vi "Get_New_Path_from_raw_data.vi"(9 "New Results File Name":string, 10 "New Results Folder Name":string, 11 "Raw data file":path) -> (2 "Does it already exist?":bool, 3 "New Spreadsheet Results File":path)   [LabVIEW 2011]
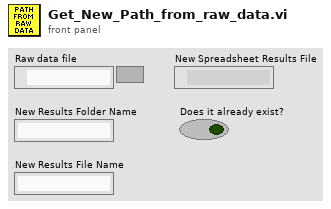
[diagram p1: front panel]
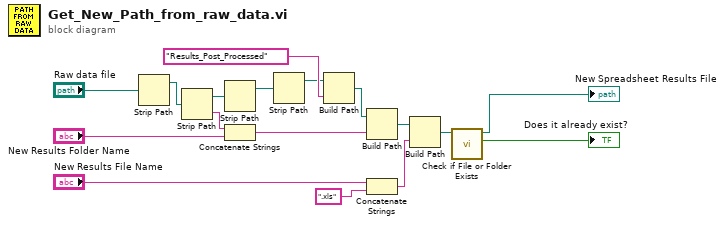
[diagram p0: block diagram]
diagram:
  n1 = Strip Path(path="Raw data file") -> (stripped path=w2:path)  [unwired: 1 out]
  n2 = Strip Path(path=w2) -> (stripped path=w4:path, name=w15:string)
  n3 = Strip Path(path=w4) -> (stripped path=w3:path)  [unwired: 1 out]
  n4 = Concatenate Strings(w15, "New Results Folder Name") -> (w14:string)
  n5 = Strip Path(path=w3) -> (stripped path=w5:path)  [unwired: 1 out]
  n6 = Build Path(base path=w5, name or relative path="Results_Post_Processed") -> (appended path=w9:path)
  n7 = Build Path(base path=w9, name or relative path=w14) -> (appended path=w12:path)
  n8 = Concatenate Strings("New Results File Name", ".xls" ("string")) -> (w16:string)
  n9 = Build Path(base path=w12, name or relative path=w16) -> (appended path=w13:path)
  n10 = call <vilib>:"Check if File or Folder Exists.vi"("path"=w13) -> ("file or folder exists?"=→"Does it already exist?":bool, "dup path"=→"New Spreadsheet Results File":path)  [unwired: 8 in, 1 out]
